vi "MU acquire Raw Data.vi"(5 "clockFrequency":dbl, 6 "AnyThread? (F)":bool, 7 "frameCycleTime":dbl, 8 "error in (no error)":errorcluster, 9 "SlaveID":u32, 10 "numberOfSamples":u64, 11 "MUhandle":u64) -> (0 "error out":errorcluster, 1 "noniusRawData":u16[](array[numeric]), 2 "masterRawData":u16[](array[numeric]), 3 "return type":u32)   [LabVIEW 2017, in "MU_3SL_interface.lvlib"]
uses:
  MU_3SL_interface.lvlib
  lib/MU_3SL_interface.dll
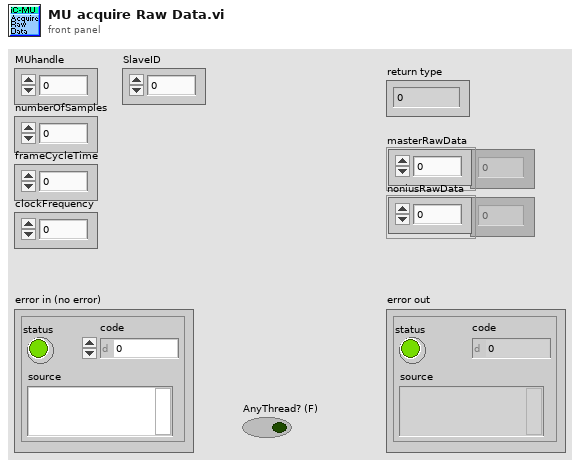
[diagram p1: front panel]
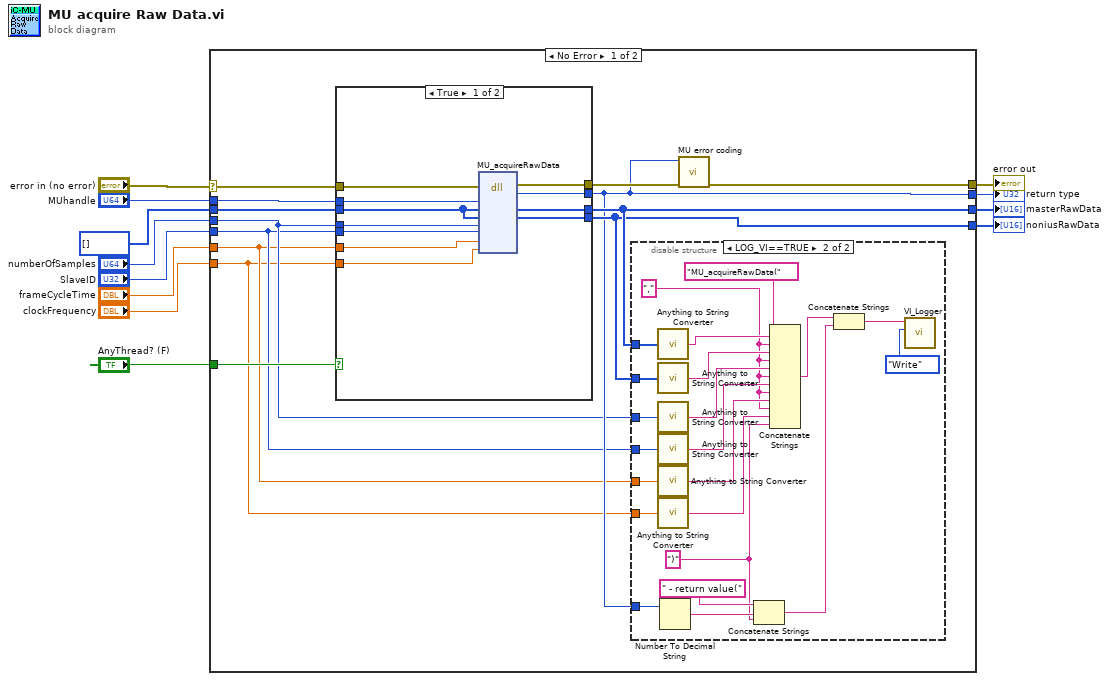
[diagram p0: block diagram]
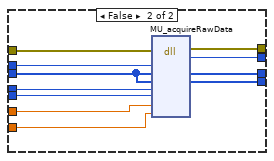
[diagram p3: hidden frame]
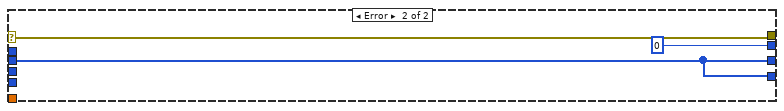
[diagram p4: hidden frame]
diagram:
  n1 = case shown="No Error" "error in (no error)" {
    selector: "error in (no error)" -> [w25 w72]
    tunnel: [w21 w72] -> w11
    tunnel: "MUhandle" -> [w24 _]
    tunnel: [w19 w70] -> w3
    tunnel: [w18 w70] -> w2
    tunnel: "numberOfSamples" -> [w16 _]
    tunnel: "SlaveID" -> [w15 _]
    tunnel: "frameCycleTime" -> [w14 _]
    tunnel: "clockFrequency" -> [w13 _]
    tunnel: [w17 u32 0 ("return type")] -> w5
    tunnel: u16[] [] ("masterRawData") -> [w23 w70]
    tunnel: "AnyThread? (F)" -> [w20 _]
    frame No Error {
      n2 = case shown="True" w20 {
        tunnel: w25 -> [w58 w69]
        tunnel: w24 -> [w57 w68]
        tunnel: [w56 w67] -> w19
        tunnel: [w55 w66] -> w18
        tunnel: w16 -> [w54 w65]
        tunnel: w15 -> [w53 w64]
        tunnel: w14 -> [w52 w63]
        tunnel: w13 -> [w51 w62]
        tunnel: w23 -> [w50 w61]
        tunnel: [w49 w60] -> w22
        tunnel: [w48 w59] -> w17
        frame True {
          n3 = dll-call lib="C:/Users/bes/AppData/Roaming/work/mu_9so/icsubmodules/soft_mu_3sl_master/lv_interface/lib/MU_3SL_interface**.*" fn="MU_acquireRawData"(error in=w58, "MUhandle"=w57, "masterRawData"=w50, "noniusRawData"=w50, "numberOfSamples"=w54, "SlaveID"=w53, "frameCycleTime"=w52, "clockFrequency"=w51) -> (error out=w49:errorcluster, "return type"=w48:u32, "masterRawData"=w56:u16[], "noniusRawData"=w55:u16[])  [unwired: 7 in, 1 out]
        }
        frame False {
          n4 = dll-call lib="C:/Users/bes/AppData/Roaming/work/mu_9so/icsubmodules/soft_mu_3sl_master/lv_interface/lib/MU_3SL_interface**.*" fn="MU_acquireRawData"(error in=w69, "MUhandle"=w68, "masterRawData"=w61, "noniusRawData"=w61, "numberOfSamples"=w65, "SlaveID"=w64, "frameCycleTime"=w63, "clockFrequency"=w62) -> (error out=w60:errorcluster, "return type"=w59:u32, "masterRawData"=w67:u16[], "noniusRawData"=w66:u16[])  [unwired: 7 in, 1 out]
        }
      }
      n5 = disable-structure shown="LOG_VI==TRUE" {
        disable-tunnel: w17 -> [_ w45]
        disable-tunnel: w19 -> [_ w40]
        disable-tunnel: w18 -> [_ w39]
        disable-tunnel: w16 -> [_ w36]
        disable-tunnel: w15 -> [_ w35]
        disable-tunnel: w14 -> [_ w34]
        disable-tunnel: w13 -> [_ w33]
        frame condition #0 {
        }
        frame condition #1 (active) {
          w26 = ")" ("string")
          w28 = "," ("string")
          n6 = call "Anything to String Converter.vi"("anything"=w40) -> ("String"=w38:string)
          n7 = call "Anything to String Converter.vi"("anything"=w39) -> ("String"=w37:string)
          n8 = call "Anything to String Converter.vi"("anything"=w36) -> ("String"=w31:string)
          n9 = call "Anything to String Converter.vi"("anything"=w35) -> ("String"=w30:string)
          n10 = call "Anything to String Converter.vi"("anything"=w34) -> ("String"=w29:string)
          n11 = call "Anything to String Converter.vi"("anything"=w33) -> ("String"=w27:string)
          n12 = Number To Decimal String(number=w45) -> (decimal integer string=w44:string)  [unwired: 1 in]
          n13 = Concatenate Strings(" - return value(" ("string"), w44, w26) -> (w43:string)
          n14 = Concatenate Strings("MU_acquireRawData(" ("Info in"), w38, w28, w37, w28, w31, w28, w30, w28, w29, w28, w27, w26) -> (w32:string)
          n15 = Concatenate Strings(w32, w43) -> (w42:string)
          n16 = call "VI_Logger.vi"("Action (Read)"=enum16{"Write", "Read"}."Write", "Info in"=w42) -> ()  [unwired: 8 in, 2 out]
        }
      }
      n17 = call "MU error coding.vi"("error in (no error)"=w22, "function return in"=w17) -> ("error out"=w21:errorcluster)  [unwired: 9 in]
    }
    frame Error {
    }
  }
  "error out" <- w11
  "masterRawData" <- w3
  "noniusRawData" <- w2
  "return type" <- w5
